vi "Load Config.vi"(8 "error in":errorcluster) -> (0 "error out":errorcluster, 3 "Zone Setup Array":T1[](array[typedef]))   [LabVIEW 2016]
doc: "Reads config file \"Sprinkler Configuration.txt\" from the app root directory and parses the information. for the Zone Setup Array.\n\nNote: Config file is expected to be found and to be in correct format."
uses:
  Controls/Zone Setup.ctl
  Controls/Zone.ctl
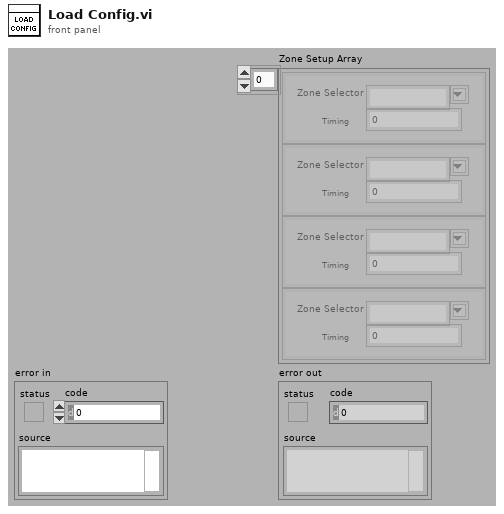
[diagram p1: front panel]
types:
  T1 = typedef "Zone Setup.ctl" = cluster{"Zone Selector":T2, "Timing":u32}
  T2 = typedef "Zone.ctl" = string
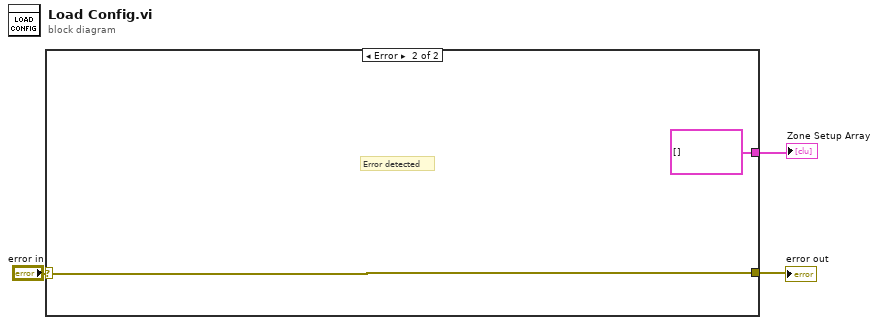
[diagram p0: block diagram]
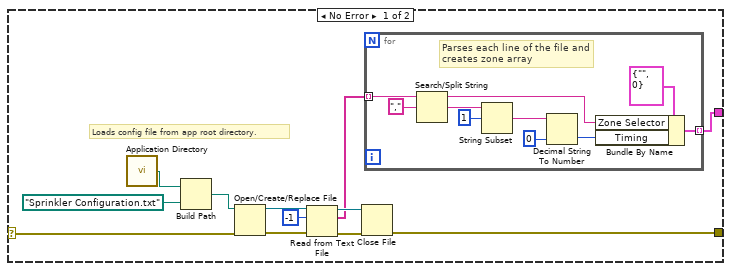
[diagram p2: hidden frame]
diagram:
  n1 = case shown="Error" "error in" {
    selector: "error in" -> [w11 w27]
    tunnel: [w10 w27] -> w2
    tunnel: [w8 T1[] []] -> w1
    frame No Error {
      # "Loads config file from app root directory."
      n2 = call <vilib>:"Application Directory.vi"() -> ("Application Directory"=w7:path)
      n3 = Build Path(base path=w7, name or relative path=path "Sprinkler Configuration.txt" ("file path (use dialog)")) -> (appended path=w5:path)
      n4 = Open/Create/Replace File(file path (use dialog)=w5, error in=w11) -> (refnum out=w14:refnum<file>, error out=w15:errorcluster)  [unwired: 4 in, 1 out]
      n5 = Read from Text File(file (use dialog)=w14, count=-1, error in=w15) -> (refnum out=w13:refnum<file>, text=w4:string[], error out=w12:errorcluster)  [unwired: 1 in, 1 out]
      n6 = Close File(refnum=w13, error in=w12) -> (error out=w10:errorcluster)  [unwired: 1 out]
      n7 = for {
        tunnel: w4 -> [w19] mode=indexing
        tunnel: [w20] -> w8 mode=indexing
        # "Parses each line of the file and \ncreates zone array"
        n8 = Search/Split String(string=w19, search string/char (-)=",") -> (substring before match=w23:string, match + rest of string=w18:string)  [unwired: 1 in, 1 out]
        n9 = String Subset(string=w18, offset (0)=1) -> (substring=w17:string)  [unwired: 1 in]
        n10 = Decimal String To Number(string=w17, default (0L)=u32 0 ("default (0 I32)")) -> (number=w22:u32)  [unwired: 1 in, 1 out]
        n11 = Bundle By Name(cluster=T1 {"Zone Selector"="", "Timing"=0} ("Zone Setup"), "Zone Selector"=w23, "Timing"=w22) -> (w20:T1)
      }
    }
    frame Error {
      # "Error detected"
    }
  }
  "error out" <- w2
  "Zone Setup Array" <- w1
